vi "Read.vi"(8 "error in (no error)":errorcluster, 11 "IP Connection in":refnum<class "IP Connection.lvclass">) -> (0 "error out":errorcluster, 1 "Function ID":u8, 2 "Stack ID":u8, 3 "IP Connection out":refnum<class "IP Connection.lvclass">, 4 "Data":string, 5 "timed out":bool)   [LabVIEW 2011, in "Tinkerforge.lvlib" / "IP Connection.lvclass"]
doc: "This VI reads a complete message."
uses:
  IP Connection.lvclass
  IP Connection.lvclass/IP Connection.ctl
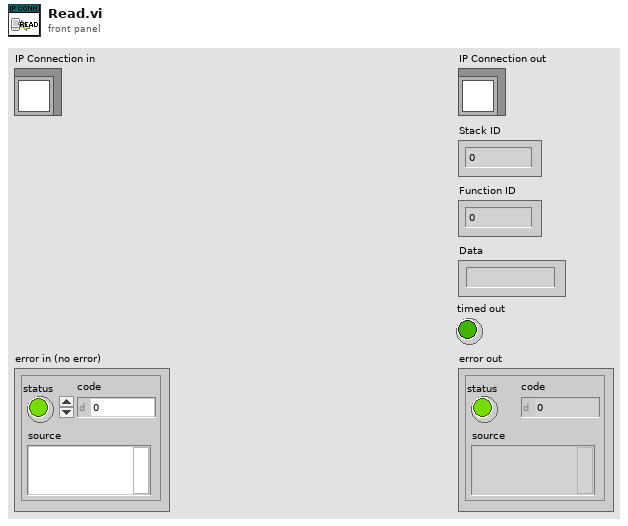
[diagram p1: front panel]
types:
  T1 = enum16{"Standard", "Buffered", "CRLF", "Immediate"}
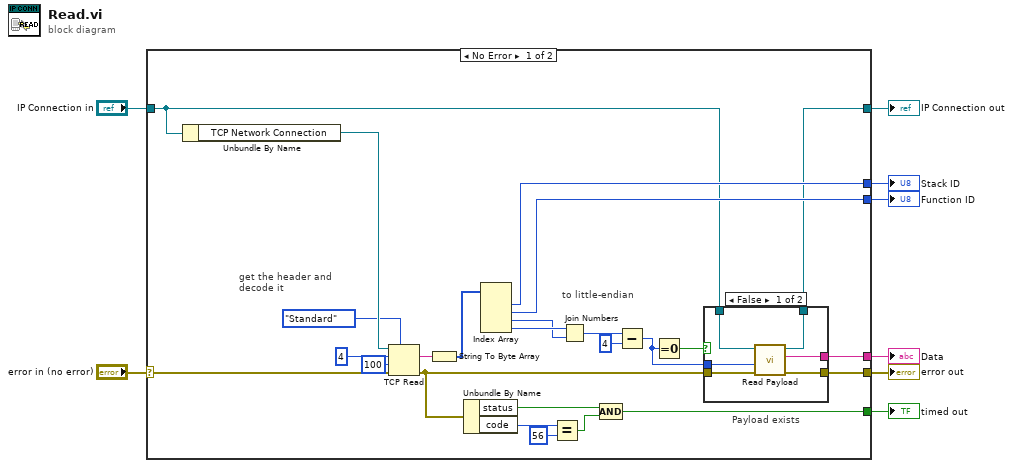
[diagram p0: block diagram]
diagram:
  n1 = case shown="No Error" "error in (no error)" {
    selector: "error in (no error)" -> [w33 w43]
    tunnel: [w21 w43] -> w7
    tunnel: [w18 w42] -> w5
    tunnel: "IP Connection in" -> [w19 w42]
    tunnel: [w27 _] -> w4
    tunnel: [w26 _] -> w3
    tunnel: [w16 _] -> w2
    tunnel: [w10 _] -> w1
    frame No Error {
      # "to little-endian"
      # "get the header and\ndecode it"
      n2 = Unbundle By Name(w19) -> ("TCP Network Connection"=w32:refnum<k5>)
      n3 = TCP Read(connection ID=w32, bytes to read=4, error in (no error)=w33, 7:T1."Standard" ("mode (standard)"), 9:100 ("timeout ms (25000)")) -> (data out=w29:string, error out=w15:errorcluster)  [unwired: 1 out]
      n4 = String To Byte Array(string=w29) -> (unsigned byte array=w28:u8[])
      n5 = Unbundle By Name(w15) -> ("status"=w11:bool, "code"=w14:i32)
      n6 = Index Array(array=w28) -> (element #1=w27:u8, element #2=w26:u8, element #3=w24:u8, element #4=w25:u8)  [unwired: 4 in]
      n7 = Equal?(x=w14, y=56) -> (x = y?=w12:bool)
      n8 = Join Numbers(hi=w25, lo=w24) -> ((hi.lo)=w23:u16)
      n9 = Compound Arithmetic op=AND(w11, w12) -> (w10:bool)
      n10 = Subtract(x=w23, y=u16 4 ("x")) -> (x-y=w20:u16)
      n11 = Equal To 0?(x=w20) -> (x = 0?=w17:bool)
      n12 = case "Payload exists" shown="False" w17 {
        tunnel: w15 -> [w39 w41]
        tunnel: [w38 w41] -> w21
        tunnel: w20 -> [w37 _]
        tunnel: w19 -> [w36 w40]
        tunnel: [w35 w40] -> w18
        tunnel: [w34 _] -> w16
        frame False {
          n13 = call "Read Payload.vi"("error in (no error)"=w39, "Payload Size"=w37, "IP Connection in"=w36) -> ("error out"=w38:errorcluster, "Data"=w34:string, "IP Connection out"=w35:refnum<class "IP Connection.lvclass">)  [unwired: 6 in]
        }
        frame True {
        }
      }
    }
    frame Error {
    }
  }
  "error out" <- w7
  "IP Connection out" <- w5
  "Stack ID" <- w4
  "Function ID" <- w3
  "Data" <- w2
  "timed out" <- w1
